vi "find_side_points.vi"(9 "corner":dbl[][](array[numeric]), 10 "X  coords array":dbl[](array[numeric]), 11 "Y coords array":dbl[](array[numeric])) -> (1 "Bottom side points":dbl[][](array[numeric]), 2 "Right side points":dbl[][](array[numeric]), 3 "Top side points":dbl[][](array[numeric]), 4 "Left side points":dbl[][](array[numeric]))   [LabVIEW 2017]
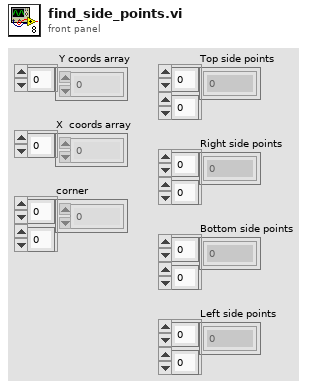
[diagram p1: front panel]
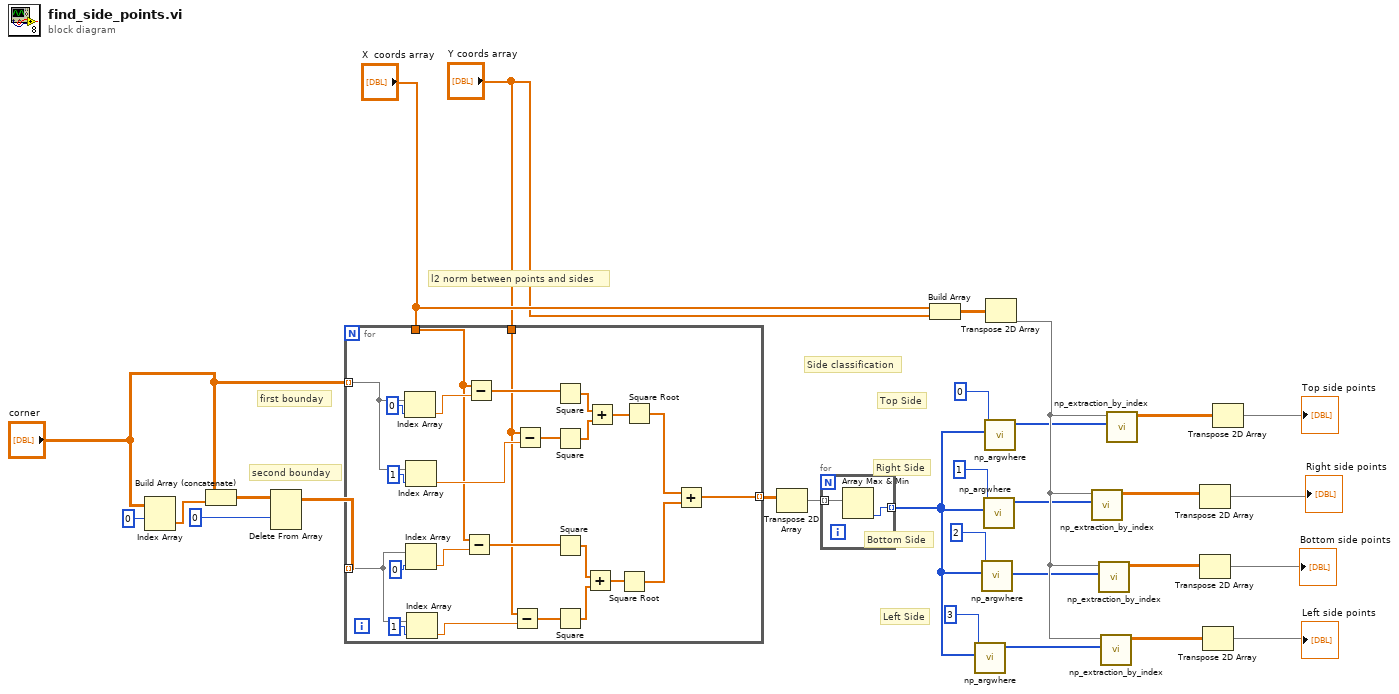
[diagram p0: block diagram]
diagram:
  # "Top Side"
  # "Left Side"
  # "Bottom Side"
  # "Right Side"
  # "l2 norm between points and sides"
  # "Side classification"
  # "first bounday"
  # "second bounday"
  n1 = Index Array "Index Array"(array="corner", index (row)=0 ("disabled index (col)")) -> (element=w10:dbl[])  [unwired: 1 in]
  n2 = Build Array (concatenate)("corner", w10) -> (w11:dbl[][])
  n3 = Delete From Array(array=w11, index (row)=0) -> (array with subset deleted=w14:dbl[][])  [unwired: 2 in, 1 out]
  n4 = for {
    tunnel: "corner" -> [w52] mode=indexing
    tunnel: w14 -> [w48] mode=indexing
    tunnel: [w32] -> w15 mode=indexing
    tunnel: "X  coords array" -> [w31]
    tunnel: "Y coords array" -> [w30]
    n5 = Index Array(array=w52, index=0) -> (element=w51:dbl)
    n6 = Index Array(array=w52, index=1) -> (element=w47:dbl)
    n7 = Index Array(array=w48, index=0) -> (element=w46:dbl)
    n8 = Index Array(array=w48, index=1) -> (element=w45:dbl)
    n9 = Subtract(x=w31, y=w46) -> (x-y=w42:dbl[])
    n10 = Subtract(x=w31, y=w51) -> (x-y=w44:dbl[])
    n11 = Subtract(x=w30, y=w45) -> (x-y=w41:dbl[])
    n12 = Subtract(x=w30, y=w47) -> (x-y=w43:dbl[])
    n13 = Square(x=w44) -> (x^2=w40:dbl[])
    n14 = Square(x=w43) -> (x^2=w39:dbl[])
    n15 = Square(x=w42) -> (x^2=w38:dbl[])
    n16 = Square(x=w41) -> (x^2=w37:dbl[])
    n17 = Add(x=w38, y=w37) -> (x+y=w35:dbl[])
    n18 = Add(x=w40, y=w39) -> (x+y=w36:dbl[])
    n19 = Square Root(x=w35) -> (sqrt(x)=w33:dbl[])
    n20 = Square Root(x=w36) -> (sqrt(x)=w34:dbl[])
    n21 = Add(x=w34, y=w33) -> (x+y=w32:dbl[])
  }
  n22 = Transpose 2D Array(2D array=w15) -> (transposed array=w16:dbl[][])
  n23 = for {
    tunnel: w16 -> [w56] mode=indexing
    tunnel: [w55] -> w24 mode=indexing
    n24 = Array Max & Min(array=w56) -> (min index (indices)=w55:i32)  [unwired: 3 out]
  }
  n25 = Build Array("X  coords array", "Y coords array") -> (w19:dbl[][])
  n26 = call "np_argwhere.vi"("Array in"=w24, "value"=3) -> ("index"=w28:i32[])  [unwired: 9 in]
  n27 = call "np_argwhere.vi"("Array in"=w24, "value"=2) -> ("index"=w27:i32[])  [unwired: 9 in]
  n28 = call "np_argwhere.vi"("Array in"=w24, "value"=1) -> ("index"=w26:i32[])  [unwired: 9 in]
  n29 = call "np_argwhere.vi"("Array in"=w24, "value"=0) -> ("index"=w25:i32[])  [unwired: 9 in]
  n30 = Transpose 2D Array(2D array=w19) -> (transposed array=w29:dbl[][])
  n31 = call "np_extraction_by_index.vi"("index array"=w26, "Array in"=w29) -> ("Array out"=w6:dbl[][])  [unwired: 9 in]
  n32 = call "np_extraction_by_index.vi"("index array"=w27, "Array in"=w29) -> ("Array out"=w4:dbl[][])  [unwired: 9 in]
  n33 = call "np_extraction_by_index.vi"("index array"=w28, "Array in"=w29) -> ("Array out"=w2:dbl[][])  [unwired: 9 in]
  n34 = call "np_extraction_by_index.vi"("index array"=w25, "Array in"=w29) -> ("Array out"=w8:dbl[][])  [unwired: 9 in]
  n35 = Transpose 2D Array(2D array=w6) -> (transposed array=→"Right side points":dbl[][])
  n36 = Transpose 2D Array(2D array=w4) -> (transposed array=→"Bottom side points":dbl[][])
  n37 = Transpose 2D Array(2D array=w2) -> (transposed array=→"Left side points":dbl[][])
  n38 = Transpose 2D Array(2D array=w8) -> (transposed array=→"Top side points":dbl[][])
